vi "Get Property by Name.vi"(8 "error in (no error)":errorcluster, 10 "Name":string, 11 "Tag in":refnum<class "Tag.lvclass">) -> (0 "error out":errorcluster, 1 "Value":variant, 2 "Found?":bool, 3 "Tag out":refnum<class "Tag.lvclass">)   [LabVIEW 2018, in "Tag Engine.lvlib" / "Tag.lvclass"]
uses:
  Tag.lvclass
  Tag.lvclass/Tag.ctl
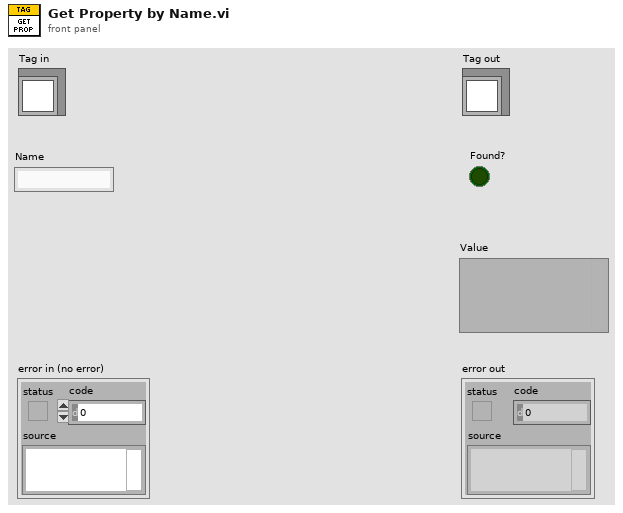
[diagram p1: front panel]
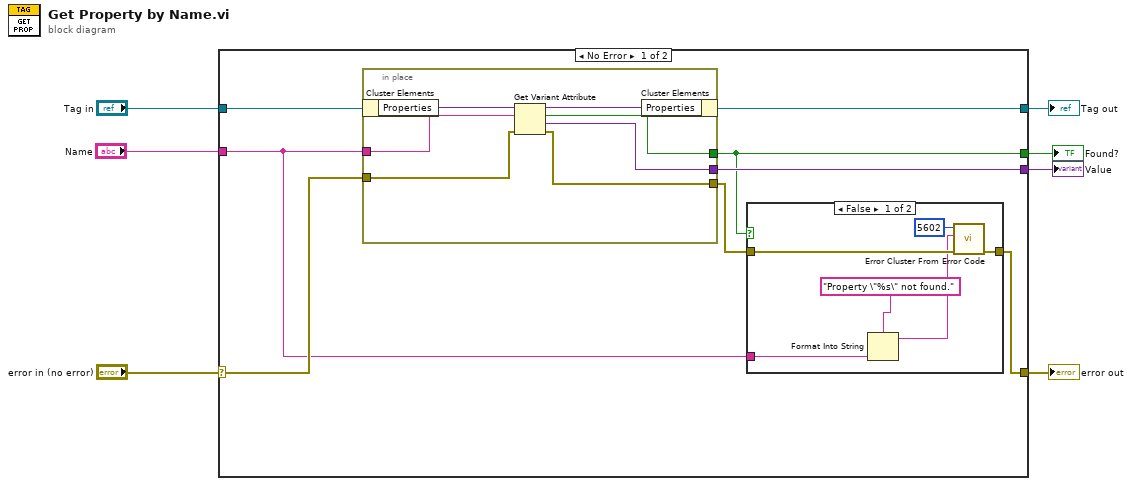
[diagram p0: block diagram]
diagram:
  n1 = case shown="No Error" "error in (no error)" {
    selector: "error in (no error)" -> [w12 w31]
    tunnel: [w8 w31] -> w6
    tunnel: [w14 w30] -> w4
    tunnel: "Tag in" -> [w15 w30]
    tunnel: "Name" -> [w10 _]
    tunnel: [w9 _] -> w2
    tunnel: [w13 _] -> w1
    frame No Error {
      n2 = in-place {
        in-place-border: w10 -> [w23]
        in-place-border: [w27] -> w9
        in-place-border: [w26] -> w13
        in-place-border: w12 -> [w25]
        in-place-border: [w24] -> w11
        n3 = in-place-cluster #1(w15) -> ("Properties"=w29:variant)
        n4 = Get Variant Attribute(Variant=w29, name=w23, error in=w25) -> (duplicate Variant=w28:variant, found=w27:bool, value=w26:variant, error out=w24:errorcluster)  [unwired: 1 in]
        n5 = in-place-cluster #1("Properties"=w28) -> (w14:refnum<class "Tag.lvclass">)
      }
      n6 = case shown="False" w9 {
        tunnel: w11 -> [w21 w22]
        tunnel: [w20 w22] -> w8
        tunnel: w10 -> [w17 _]
        frame False {
          n7 = Format Into String(format string="Property \"%s\" not found.", w17) -> (resulting string=w16:string)  [unwired: 2 in, 1 out]
          n8 = call <vilib>:"Error Cluster From Error Code.vi"("error in (no error)"=w21, "error message (\"\")"=w16, "error code (0)"=5602) -> ("error out"=w20:errorcluster)  [unwired: 6 in]
        }
        frame True {
        }
      }
    }
    frame Error {
    }
  }
  "error out" <- w6
  "Tag out" <- w4
  "Found?" <- w2
  "Value" <- w1
